vi "Auswertung Registerkarte.vi"(0 "GObject (Eingang)":refnum<vi>, 5 "ClassID":u32, 7 "all rows":string[][](array[string]), 9 "Sprachauswahl":u32, 11 "Fehler (Eingang, kein Fehler)":errorcluster) -> (4 "Clusterelemente":refnum<vi>[](array[refnum]), 15 "error out":errorcluster caption="Fehler (Ausgang)")   [LabVIEW 2015, in "Sprachverwaltung.lvlib"]
uses:
  Sprachverwaltung.lvlib
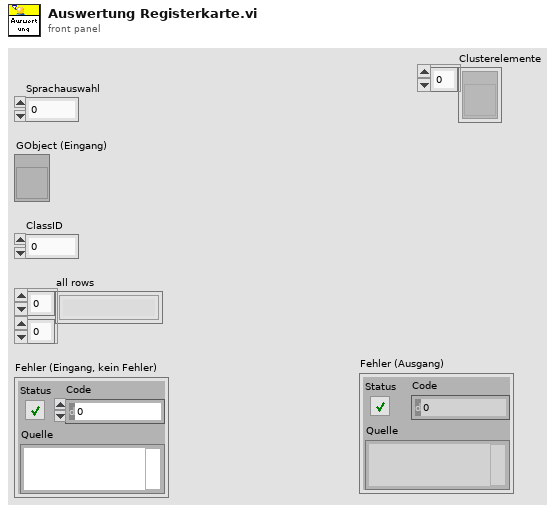
[diagram p1: front panel]
types:
  T1 = typedef "LVStringsAndValuesArrayTypeDef.ctl" = cluster{"String":string, "Value":ext}[]
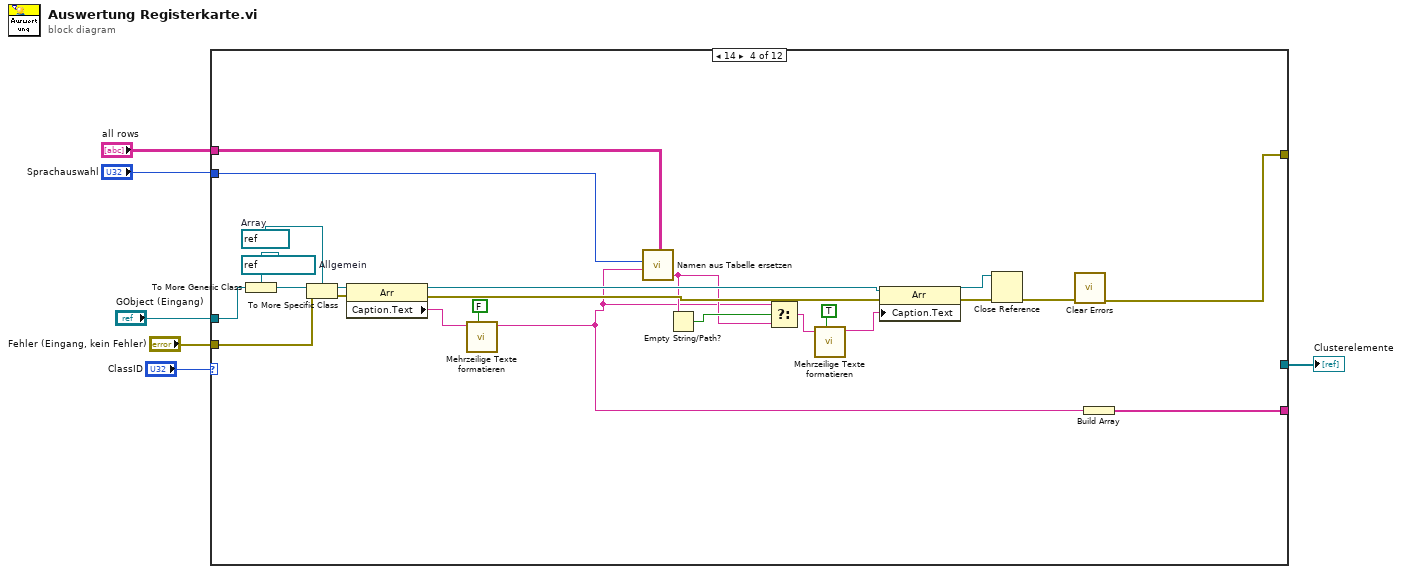
[diagram p0: block diagram]
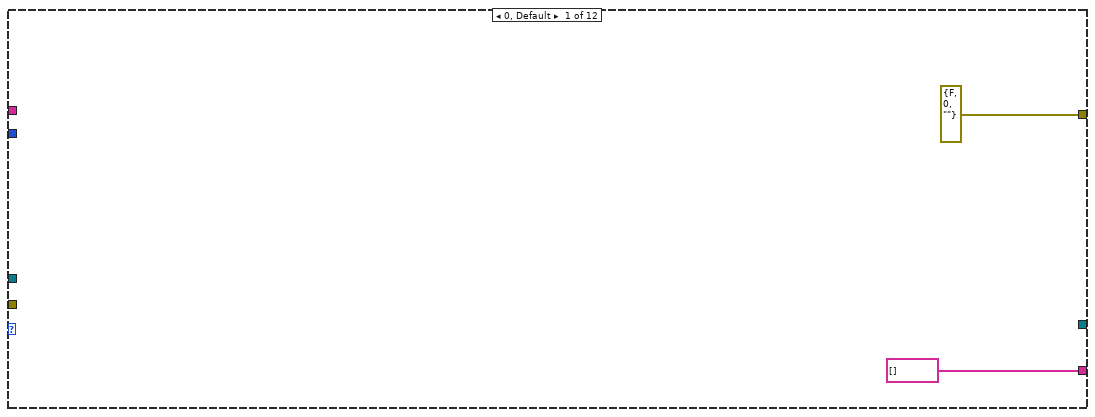
[diagram p2: hidden frame]
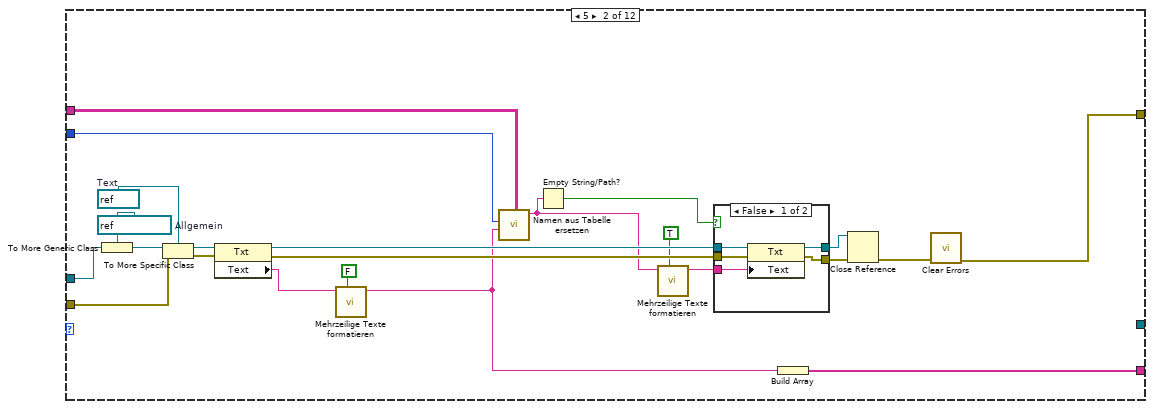
[diagram p3: hidden frame]
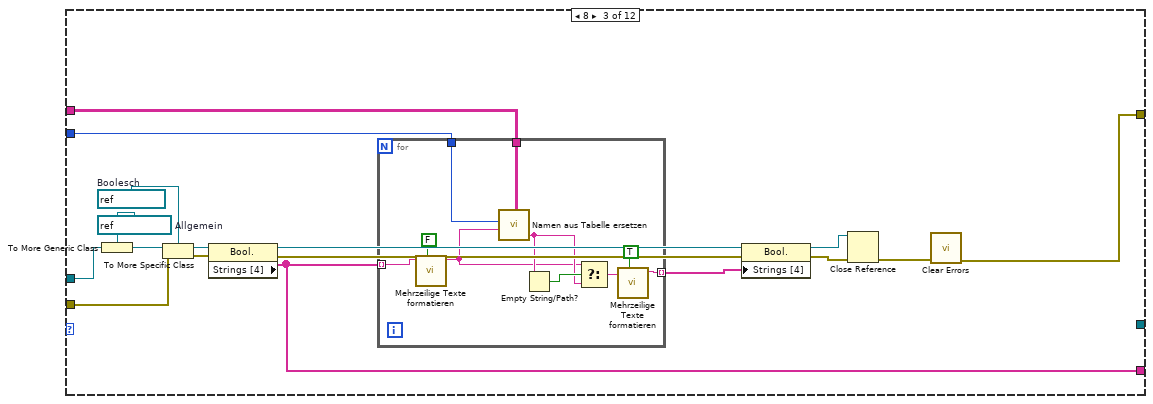
[diagram p5: hidden frame]
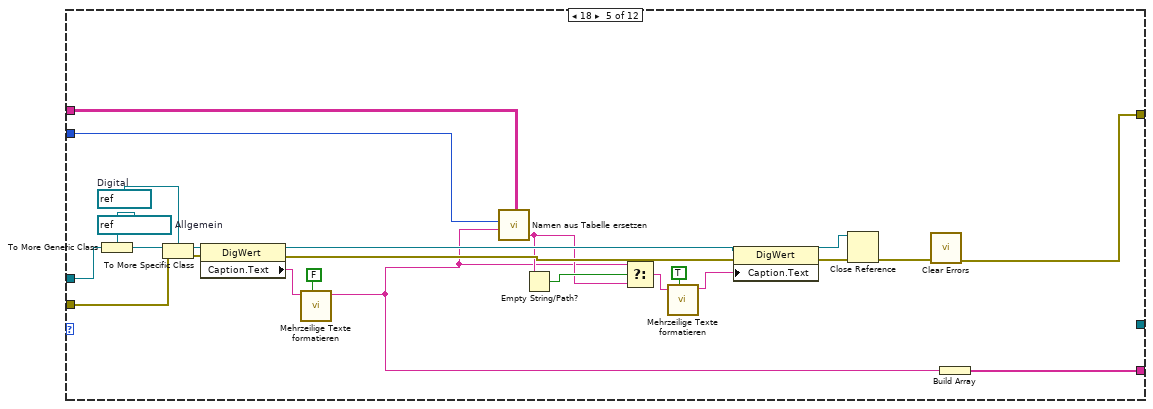
[diagram p6: hidden frame]
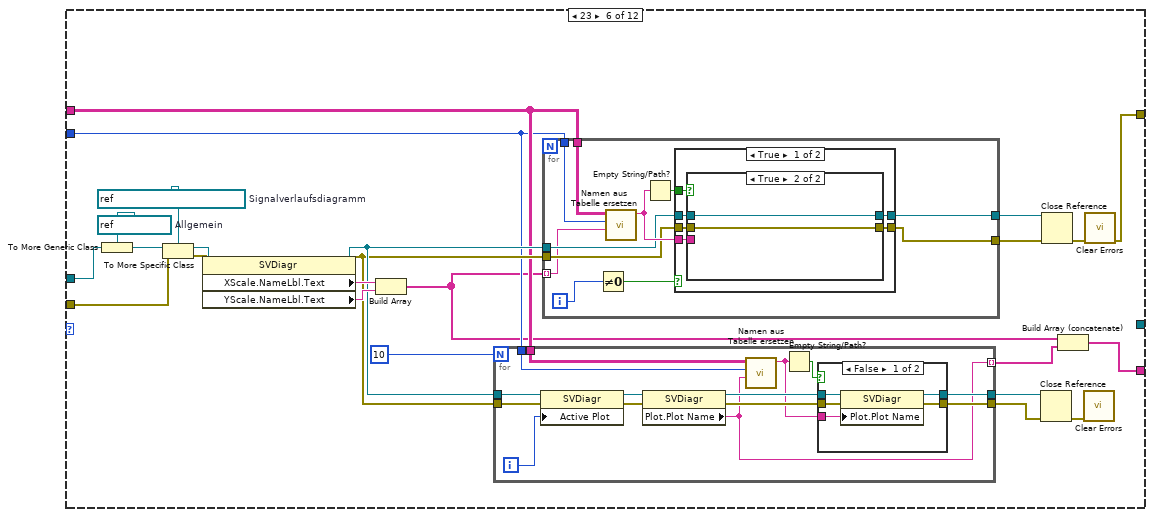
[diagram p7: hidden frame]
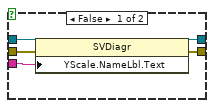
[diagram p9: hidden frame]
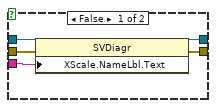
[diagram p11: hidden frame]
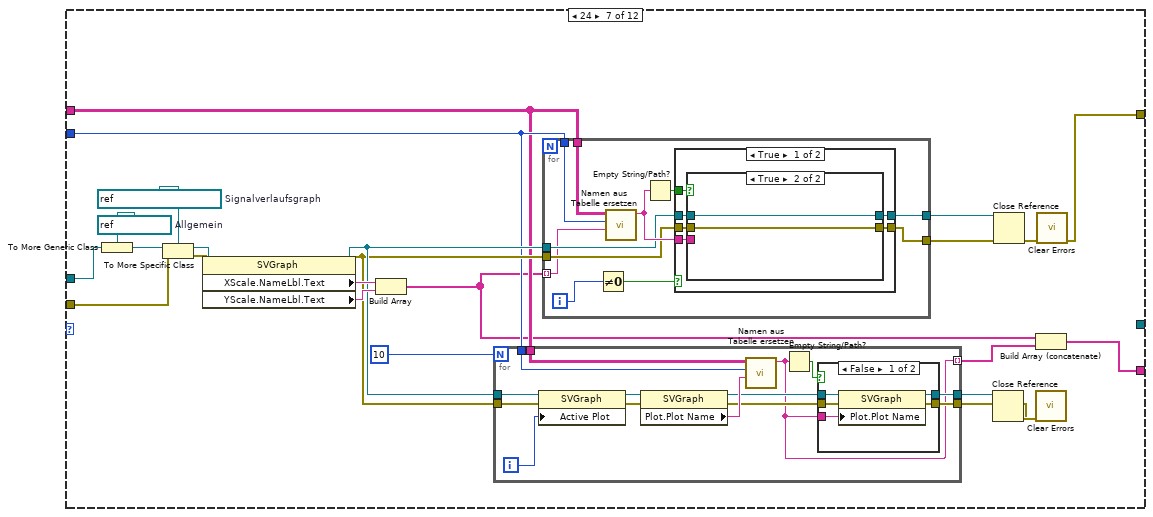
[diagram p12: hidden frame]
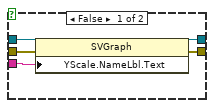
[diagram p14: hidden frame]
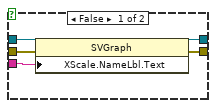
[diagram p16: hidden frame]
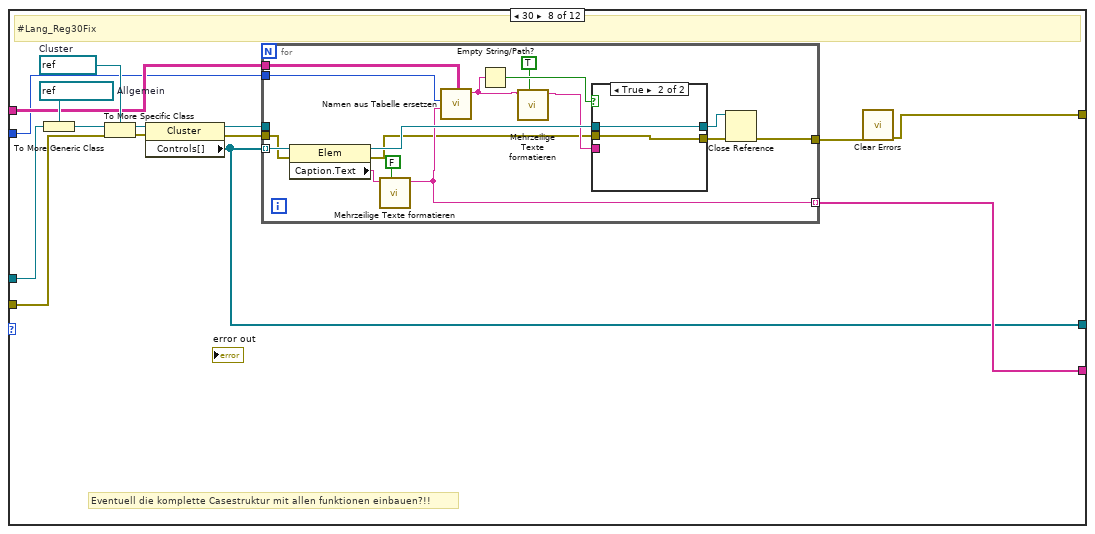
[diagram p17: hidden frame]
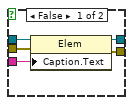
[diagram p18: hidden frame]
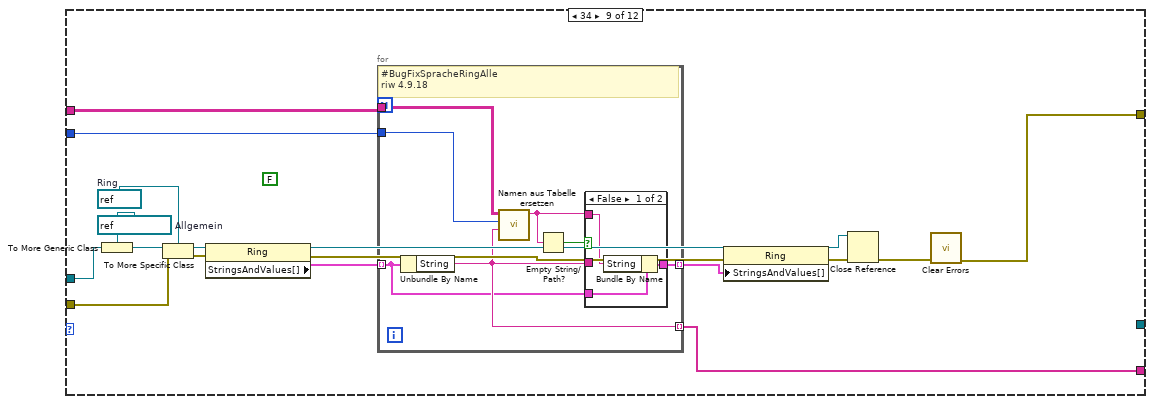
[diagram p19: hidden frame]
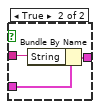
[diagram p20: hidden frame]
diagram:
  n1 = case shown="14" "ClassID" {
    tunnel: "GObject (Eingang)" -> [_ w31 w55 w89 w113 w137 w219 w292 w333 w372 w386 w443]
    tunnel: "Fehler (Eingang, kein Fehler)" -> [_ w28 w52 w86 w110 w134 w216 w289 w330 w369 w387 w440]
    tunnel: "all rows" -> [_ w24 w50 w82 w106 w122 w200 w285 w325 w361 w389 w428]
    tunnel: "Sprachauswahl" -> [_ w17 w49 w81 w105 w121 w204 w284 w324 w360 w388 w420]
    tunnel: [string[] [] ("Strings [4]") w16 w42 w74 w98 w115 w197 w283 w318 w348 w390 w422] -> _
    tunnel: [errorcluster {"status"=FALSE, "code"=0, "source"=""} ("error out") w15 w41 w75 w99 w114 w196 w279 w317 w347 w385 w421] -> _
    tunnel: [_ _ _ _ _ _ _ w278 _ _ _ _] -> w1
    frame 0, Default {
    }
    frame 5 {
      w27 = refnum<vi> refnum  # Text
      w30 = refnum<vi> refnum  # Allgemein
      n2 = To More Generic Class(target class=w30, reference=w31) -> (generic class reference=w29:refnum<vi>)
      n3 = To More Specific Class(target class=w27, reference=w29, error in=w28) -> (specific class reference=w26:refnum<vi>, error out=w25:errorcluster)
      n4 = property class="Txt"(reference=w26, error in=w25) -> (reference out=w22:refnum<vi>, error out=w23:errorcluster, "Text"=w14:string)
      n5 = call "Mehrzeilige Texte formatieren.vi"("Zurück formatieren"=FALSE, "string"=w14) -> ("result string"=w13:string)  [unwired: 9 in]
      n6 = call "Namen aus Tabelle ersetzen.vi"("Regulärer Ausdruck"=w13, "Sprachauswahl"=w17, "Tabelle"=w24) -> ("Übersetzung"=w10:string)  [unwired: 8 in]
      n7 = Empty String/Path?(string/path=w10) -> (empty?=w18:bool)
      n8 = call "Mehrzeilige Texte formatieren.vi"("Zurück formatieren"=TRUE, "string"=w10) -> ("result string"=w9:string)  [unwired: 9 in]
      n9 = case shown="False" w18 {
        tunnel: w23 -> [w36 w37]
        tunnel: w22 -> [w35 w38]
        tunnel: w9 -> [w34 _]
        tunnel: [w33 w37] -> w21
        tunnel: [w32 w38] -> w20
        frame False {
          n10 = property class="Txt"(reference=w35, error in=w36, "Text"=w34) -> (reference out=w32:refnum<vi>, error out=w33:errorcluster)
        }
        frame True {
        }
      }
      n11 = Build Array(w13) -> (w16:string[])
      n12 = Close Reference(reference=w20, error in (no error)=w21) -> (error out=w19:errorcluster)
      n13 = call <vilib>:"Clear Errors.vi"("error in (no error)"=w19) -> ("error out"=w15:errorcluster)  [unwired: 5 in, 1 out]
    }
    frame 8 {
      w51 = refnum<vi> refnum  # Boolesch
      w54 = refnum<vi> refnum  # Allgemein
      n14 = To More Generic Class(target class=w54, reference=w55) -> (generic class reference=w53:refnum<vi>)
      n15 = To More Specific Class(target class=w51, reference=w53, error in=w52) -> (specific class reference=w39:refnum<vi>, error out=w40:errorcluster)
      n16 = property class="Bool."(reference=w39, error in=w40) -> (reference out=w47:refnum<vi>, error out=w48:errorcluster, "Strings [4]"=w42:string[])
      n17 = for {
        tunnel: w42 -> [w60] mode=indexing
        tunnel: w50 -> [w65]
        tunnel: w49 -> [w64]
        tunnel: [w56] -> w43 mode=indexing
        n18 = call "Mehrzeilige Texte formatieren.vi"("Zurück formatieren"=FALSE, "string"=w60) -> ("result string"=w59:string)  [unwired: 9 in]
        n19 = call "Namen aus Tabelle ersetzen.vi"("Regulärer Ausdruck"=w59, "Sprachauswahl"=w64, "Tabelle"=w65) -> ("Übersetzung"=w62:string)  [unwired: 8 in]
        n20 = Empty String/Path?(string/path=w62) -> (empty?=w63:bool)
        n21 = Select(t=w59, s=w63, f=w62) -> (s? t:f=w57:string)
        n22 = call "Mehrzeilige Texte formatieren.vi"("Zurück formatieren"=TRUE, "string"=w57) -> ("result string"=w56:string)  [unwired: 9 in]
      }
      n23 = property class="Bool."(reference=w47, error in=w48, "Strings [4]"=w43) -> (reference out=w45:refnum<vi>, error out=w46:errorcluster)
      n24 = Close Reference(reference=w45, error in (no error)=w46) -> (error out=w44:errorcluster)
      n25 = call <vilib>:"Clear Errors.vi"("error in (no error)"=w44) -> ("error out"=w41:errorcluster)  [unwired: 5 in, 1 out]
    }
    frame 14 {
      w85 = refnum<vi> refnum  # Array
      w88 = refnum<vi> refnum  # Allgemein
      n26 = To More Generic Class(target class=w88, reference=w89) -> (generic class reference=w87:refnum<vi>)
      n27 = To More Specific Class(target class=w85, reference=w87, error in=w86) -> (specific class reference=w84:refnum<vi>, error out=w83:errorcluster)
      n28 = property class="Arr"(reference=w84, error in=w83) -> (reference out=w79:refnum<vi>, error out=w80:errorcluster, "Caption.Text"=w70:string)
      n29 = call "Mehrzeilige Texte formatieren.vi"("Zurück formatieren"=FALSE, "string"=w70) -> ("result string"=w69:string)  [unwired: 9 in]
      n30 = call "Namen aus Tabelle ersetzen.vi"("Regulärer Ausdruck"=w69, "Sprachauswahl"=w81, "Tabelle"=w82) -> ("Übersetzung"=w72:string)  [unwired: 8 in]
      n31 = Empty String/Path?(string/path=w72) -> (empty?=w73:bool)
      n32 = Select(t=w69, s=w73, f=w72) -> (s? t:f=w67:string)
      n33 = call "Mehrzeilige Texte formatieren.vi"("Zurück formatieren"=TRUE, "string"=w67) -> ("result string"=w66:string)  [unwired: 9 in]
      n34 = property class="Arr"(reference=w79, error in=w80, "Caption.Text"=w66) -> (reference out=w77:refnum<vi>, error out=w78:errorcluster)
      n35 = Close Reference(reference=w77, error in (no error)=w78) -> (error out=w76:errorcluster)
      n36 = call <vilib>:"Clear Errors.vi"("error in (no error)"=w76) -> ("error out"=w75:errorcluster)  [unwired: 5 in, 1 out]
      n37 = Build Array(w69) -> (w74:string[])
    }
    frame 18 {
      w109 = refnum<vi> refnum  # Digital
      w112 = refnum<vi> refnum  # Allgemein
      n38 = To More Generic Class(target class=w112, reference=w113) -> (generic class reference=w111:refnum<vi>)
      n39 = To More Specific Class(target class=w109, reference=w111, error in=w110) -> (specific class reference=w108:refnum<vi>, error out=w107:errorcluster)
      n40 = property class="DigWert"(reference=w108, error in=w107) -> (reference out=w103:refnum<vi>, error out=w104:errorcluster, "Caption.Text"=w94:string)
      n41 = call "Mehrzeilige Texte formatieren.vi"("Zurück formatieren"=FALSE, "string"=w94) -> ("result string"=w93:string)  [unwired: 9 in]
      n42 = call "Namen aus Tabelle ersetzen.vi"("Regulärer Ausdruck"=w93, "Sprachauswahl"=w105, "Tabelle"=w106) -> ("Übersetzung"=w96:string)  [unwired: 8 in]
      n43 = Empty String/Path?(string/path=w96) -> (empty?=w97:bool)
      n44 = Select(t=w93, s=w97, f=w96) -> (s? t:f=w91:string)
      n45 = call "Mehrzeilige Texte formatieren.vi"("Zurück formatieren"=TRUE, "string"=w91) -> ("result string"=w90:string)  [unwired: 9 in]
      n46 = property class="DigWert"(reference=w103, error in=w104, "Caption.Text"=w90) -> (reference out=w101:refnum<vi>, error out=w102:errorcluster)
      n47 = Close Reference(reference=w101, error in (no error)=w102) -> (error out=w100:errorcluster)
      n48 = call <vilib>:"Clear Errors.vi"("error in (no error)"=w100) -> ("error out"=w99:errorcluster)  [unwired: 5 in, 1 out]
      n49 = Build Array(w93) -> (w98:string[])
    }
    frame 23 {
      w133 = refnum<vi> refnum  # Signalverlaufsdiagramm
      w136 = refnum<vi> refnum  # Allgemein
      n50 = To More Generic Class(target class=w136, reference=w137) -> (generic class reference=w135:refnum<vi>)
      n51 = To More Specific Class(target class=w133, reference=w135, error in=w134) -> (specific class reference=w132:refnum<vi>, error out=w131:errorcluster)
      n52 = property class="SVDiagr"(reference=w132, error in=w131) -> (reference out=w127:refnum<vi>, error out=w125:errorcluster, "XScale.NameLbl.Text"=w130:string, "YScale.NameLbl.Text"=w129:string)
      n53 = Build Array(w130, w129) -> (w117:string[])
      n54 = for {
        N: 10 -> [_]
        tunnel: w127 -> [w151]
        tunnel: w125 -> [w147]
        tunnel: w122 -> [w146]
        tunnel: w121 -> [w145]
        tunnel: [w141] -> w119
        tunnel: [w140] -> w118
        tunnel: [w138] -> w116 mode=indexing
        i -> [w150]
        n55 = property class="SVDiagr"(reference=w151, error in=w147, "Active Plot"=w150) -> (reference out=w149:refnum<vi>, error out=w148:errorcluster)
        n56 = property class="SVDiagr"(reference=w149, error in=w148) -> (reference out=w144:refnum<vi>, error out=w143:errorcluster, "Plot.Plot Name"=w138:string)
        n57 = call "Namen aus Tabelle ersetzen.vi"("Regulärer Ausdruck"=w138, "Sprachauswahl"=w145, "Tabelle"=w146) -> ("Übersetzung"=w139:string)  [unwired: 8 in]
        n58 = Empty String/Path?(string/path=w139) -> (empty?=w142:bool)
        n59 = case shown="False" w142 {
          tunnel: w144 -> [w156 w158]
          tunnel: w143 -> [w155 w157]
          tunnel: [w154 w158] -> w141
          tunnel: [w153 w157] -> w140
          tunnel: w139 -> [w152 _]
          frame False {
            n60 = property class="SVDiagr"(reference=w156, error in=w155, "Plot.Plot Name"=w152) -> (reference out=w154:refnum<vi>, error out=w153:errorcluster)
          }
          frame True {
          }
        }
      }
      n61 = for {
        tunnel: w122 -> [w169]
        tunnel: w121 -> [w160]
        tunnel: w117 -> [w159] mode=indexing
        tunnel: w127 -> [w164]
        tunnel: w125 -> [w163]
        tunnel: [w162] -> w124
        tunnel: [w161] -> w123
        i -> [w166]
        n62 = Not Equal To 0?(x=w166) -> (x != 0?=w165:bool)
        n63 = call "Namen aus Tabelle ersetzen.vi"("Regulärer Ausdruck"=w159, "Sprachauswahl"=w160, "Tabelle"=w169) -> ("Übersetzung"=w167:string)  [unwired: 8 in]
        n64 = Empty String/Path?(string/path=w167) -> (empty?=w168:bool)
        n65 = case shown="True" w165 {
          tunnel: w168 -> [w175 w188]
          tunnel: w167 -> [w174 w187]
          tunnel: w164 -> [w173 w186]
          tunnel: w163 -> [w172 w185]
          tunnel: [w171 w183] -> w161
          tunnel: [w170 w184] -> w162
          frame True {
            n66 = case shown="True" w175 {
              tunnel: w172 -> [w180 w181]
              tunnel: w173 -> [w179 w182]
              tunnel: [w178 w181] -> w171
              tunnel: [w177 w182] -> w170
              tunnel: w174 -> [w176 _]
              frame False {
                n67 = property class="SVDiagr"(reference=w179, error in=w180, "YScale.NameLbl.Text"=w176) -> (reference out=w177:refnum<vi>, error out=w178:errorcluster)
              }
              frame True {
              }
            }
          }
          frame False {
            n68 = case shown="True" w188 {
              tunnel: w185 -> [w193 w194]
              tunnel: w186 -> [w192 w195]
              tunnel: [w191 w194] -> w183
              tunnel: [w190 w195] -> w184
              tunnel: w187 -> [w189 _]
              frame False {
                n69 = property class="SVDiagr"(reference=w192, error in=w193, "XScale.NameLbl.Text"=w189) -> (reference out=w190:refnum<vi>, error out=w191:errorcluster)
              }
              frame True {
              }
            }
          }
        }
      }
      n70 = Close Reference(reference=w119, error in (no error)=w118) -> (error out=w120:errorcluster)
      n71 = Close Reference(reference=w124, error in (no error)=w123) -> (error out=w128:errorcluster)
      n72 = Build Array (concatenate)(w117, w116) -> (w115:string[])
      n73 = call <vilib>:"Clear Errors.vi"("error in (no error)"=w120) -> ()  [unwired: 5 in, 2 out]
      n74 = call <vilib>:"Clear Errors.vi"("error in (no error)"=w128) -> ("error out"=w114:errorcluster)  [unwired: 5 in, 1 out]
    }
    frame 24 {
      w215 = refnum<vi> refnum  # Signalverlaufsgraph
      w218 = refnum<vi> refnum  # Allgemein
      n75 = To More Generic Class(target class=w218, reference=w219) -> (generic class reference=w217:refnum<vi>)
      n76 = To More Specific Class(target class=w215, reference=w217, error in=w216) -> (specific class reference=w214:refnum<vi>, error out=w213:errorcluster)
      n77 = property class="SVGraph"(reference=w214, error in=w213) -> (reference out=w209:refnum<vi>, error out=w207:errorcluster, "XScale.NameLbl.Text"=w212:string, "YScale.NameLbl.Text"=w211:string)
      n78 = Build Array(w212, w211) -> (w199:string[])
      n79 = for {
        N: 10 -> [_]
        tunnel: w209 -> [w233]
        tunnel: w207 -> [w229]
        tunnel: w200 -> [w228]
        tunnel: w204 -> [w227]
        tunnel: [w222] -> w202
        tunnel: [w221] -> w201
        tunnel: [w220] -> w198 mode=indexing
        i -> [w232]
        n80 = property class="SVGraph"(reference=w233, error in=w229, "Active Plot"=w232) -> (reference out=w231:refnum<vi>, error out=w230:errorcluster)
        n81 = property class="SVGraph"(reference=w231, error in=w230) -> (reference out=w225:refnum<vi>, error out=w224:errorcluster, "Plot.Plot Name"=w226:string)
        n82 = call "Namen aus Tabelle ersetzen.vi"("Regulärer Ausdruck"=w226, "Sprachauswahl"=w227, "Tabelle"=w228) -> ("Übersetzung"=w220:string)  [unwired: 8 in]
        n83 = Empty String/Path?(string/path=w220) -> (empty?=w223:bool)
        n84 = case shown="False" w223 {
          tunnel: w225 -> [w238 w240]
          tunnel: w224 -> [w237 w239]
          tunnel: [w236 w240] -> w222
          tunnel: [w235 w239] -> w221
          tunnel: w220 -> [w234 _]
          frame False {
            n85 = property class="SVGraph"(reference=w238, error in=w237, "Plot.Plot Name"=w234) -> (reference out=w236:refnum<vi>, error out=w235:errorcluster)
          }
          frame True {
          }
        }
      }
      n86 = for {
        tunnel: w200 -> [w251]
        tunnel: w204 -> [w242]
        tunnel: w199 -> [w241] mode=indexing
        tunnel: w209 -> [w246]
        tunnel: w207 -> [w245]
        tunnel: [w244] -> w206
        tunnel: [w243] -> w205
        i -> [w248]
        n87 = Not Equal To 0?(x=w248) -> (x != 0?=w247:bool)
        n88 = call "Namen aus Tabelle ersetzen.vi"("Regulärer Ausdruck"=w241, "Sprachauswahl"=w242, "Tabelle"=w251) -> ("Übersetzung"=w249:string)  [unwired: 8 in]
        n89 = Empty String/Path?(string/path=w249) -> (empty?=w250:bool)
        n90 = case shown="True" w247 {
          tunnel: w250 -> [w257 w270]
          tunnel: w249 -> [w256 w269]
          tunnel: w246 -> [w255 w268]
          tunnel: w245 -> [w254 w267]
          tunnel: [w253 w265] -> w243
          tunnel: [w252 w266] -> w244
          frame True {
            n91 = case shown="True" w257 {
              tunnel: w254 -> [w262 w263]
              tunnel: w255 -> [w261 w264]
              tunnel: [w260 w263] -> w253
              tunnel: [w259 w264] -> w252
              tunnel: w256 -> [w258 _]
              frame False {
                n92 = property class="SVGraph"(reference=w261, error in=w262, "YScale.NameLbl.Text"=w258) -> (reference out=w259:refnum<vi>, error out=w260:errorcluster)
              }
              frame True {
              }
            }
          }
          frame False {
            n93 = case shown="True" w270 {
              tunnel: w267 -> [w275 w276]
              tunnel: w268 -> [w274 w277]
              tunnel: [w273 w276] -> w265
              tunnel: [w272 w277] -> w266
              tunnel: w269 -> [w271 _]
              frame False {
                n94 = property class="SVGraph"(reference=w274, error in=w275, "XScale.NameLbl.Text"=w271) -> (reference out=w272:refnum<vi>, error out=w273:errorcluster)
              }
              frame True {
              }
            }
          }
        }
      }
      n95 = Close Reference(reference=w202, error in (no error)=w201) -> (error out=w203:errorcluster)
      n96 = Close Reference(reference=w206, error in (no error)=w205) -> (error out=w210:errorcluster)
      n97 = Build Array (concatenate)(w199, w198) -> (w197:string[])
      n98 = call <vilib>:"Clear Errors.vi"("error in (no error)"=w203) -> ()  [unwired: 5 in, 2 out]
      n99 = call <vilib>:"Clear Errors.vi"("error in (no error)"=w210) -> ("error out"=w196:errorcluster)  [unwired: 5 in, 1 out]
    }
    frame 30 {
      w288 = refnum<vi> refnum  # Cluster
      w291 = refnum<vi> refnum  # Allgemein
      # "Eventuell die komplette Casestruktur mit allen funktionen einbauen?!!"
      # "#Lang_Reg30Fix"
      n100 = To More Generic Class(target class=w291, reference=w292) -> (generic class reference=w290:refnum<vi>)
      n101 = To More Specific Class(target class=w288, reference=w290, error in=w289) -> (specific class reference=w287:refnum<vi>, error out=w286:errorcluster)
      n102 = property class="Cluster"(reference=w287, error in=w286) -> (reference out=w282:refnum<vi>, error out=w281:errorcluster, "Controls[]"=w278:refnum<vi>[])
      n103 = for {
        tunnel: w285 -> [w308]
        tunnel: w281 -> [w294]
        tunnel: w282 -> [_]
        tunnel: w284 -> [w304]
        tunnel: w278 -> [w303] mode=indexing
        tunnel: [w297] -> w283 mode=indexing
        tunnel: [w301] -> w280
        n104 = property class="Elem"(reference=w303, error in=w294) -> (reference out=w302:refnum<vi>, error out=w293:errorcluster, "Caption.Text"=w298:string)
        n105 = call "Mehrzeilige Texte formatieren.vi"("Zurück formatieren"=FALSE, "string"=w298) -> ("result string"=w297:string)  [unwired: 9 in]
        n106 = call "Namen aus Tabelle ersetzen.vi"("Regulärer Ausdruck"=w297, "Sprachauswahl"=w304, "Tabelle"=w308) -> ("Übersetzung"=w296:string)  [unwired: 8 in]
        n107 = Empty String/Path?(string/path=w296) -> (empty?=w305:bool)
        n108 = call "Mehrzeilige Texte formatieren.vi"("Zurück formatieren"=TRUE, "string"=w296) -> ("result string"=w295:string)  [unwired: 9 in]
        n109 = case shown="True" w305 {
          tunnel: w293 -> [w313 w314]
          tunnel: w302 -> [w312 w315]
          tunnel: w295 -> [w311 _]
          tunnel: [w310 w314] -> w307
          tunnel: [w309 w315] -> w306
          frame False {
            n110 = property class="Elem"(reference=w312, error in=w313, "Caption.Text"=w311) -> (reference out=w309:refnum<vi>, error out=w310:errorcluster)
          }
          frame True {
          }
        }
        n111 = Close Reference(reference=w306, error in (no error)=w307) -> (error out=w301:errorcluster)
      }
      n112 = call <vilib>:"Clear Errors.vi"("error in (no error)"=w280) -> ("error out"=w279:errorcluster)  [unwired: 5 in, 1 out]
    }
    frame 34 {
      (unwired) FALSE
      w329 = refnum<vi> refnum  # Ring
      w332 = refnum<vi> refnum  # Allgemein
      n113 = To More Generic Class(target class=w332, reference=w333) -> (generic class reference=w331:refnum<vi>)
      n114 = To More Specific Class(target class=w329, reference=w331, error in=w330) -> (specific class reference=w328:refnum<vi>, error out=w327:errorcluster)
      n115 = property class="Ring"(reference=w328, error in=w327) -> (reference out=w322:refnum<vi>, error out=w323:errorcluster, "StringsAndValues[]"=w326:T1)
      n116 = for {
        tunnel: w326 -> [w335] mode=indexing
        tunnel: w325 -> [w340]
        tunnel: w324 -> [w339]
        tunnel: [w336] -> w318 mode=indexing
        tunnel: [w334] -> w316 mode=indexing
        # "#BugFixSpracheRingAlle\nriw 4.9.18"
        n117 = Unbundle By Name(w335) -> ("String"=w336:string)
        n118 = call "Namen aus Tabelle ersetzen.vi"("Regulärer Ausdruck"=w336, "Sprachauswahl"=w339, "Tabelle"=w340) -> ("Übersetzung"=w337:string)  [unwired: 8 in]
        n119 = Empty String/Path?(string/path=w337) -> (empty?=w338:bool)
        n120 = case shown="False" w338 {
          tunnel: w335 -> [w343 w346]
          tunnel: w337 -> [w342 _]
          tunnel: [w341 w345] -> w334
          tunnel: w336 -> [_ w344]
          frame False {
            n121 = Bundle By Name(cluster=w343, "String"=w342) -> (w341:cluster{"String":string, "Value":ext})
          }
          frame True {
            n122 = Bundle By Name(cluster=w346, "String"=w344) -> (w345:cluster{"String":string, "Value":ext})
          }
        }
      }
      n123 = property class="Ring"(reference=w322, error in=w323, "StringsAndValues[]"=w316) -> (reference out=w320:refnum<vi>, error out=w321:errorcluster)
      n124 = Close Reference(reference=w320, error in (no error)=w321) -> (error out=w319:errorcluster)
      n125 = call <vilib>:"Clear Errors.vi"("error in (no error)"=w319) -> ("error out"=w317:errorcluster)  [unwired: 5 in, 1 out]
    }
    frame 46 {
      w368 = refnum<vi> refnum  # MehrspaltigesListenfeld
      w371 = refnum<vi> refnum  # Allgemein
      # "Eventuell die komplette Casestruktur mit allen funktionen einbauen?!!"
      n126 = To More Generic Class(target class=w371, reference=w372) -> (generic class reference=w370:refnum<vi>)
      n127 = To More Specific Class(target class=w368, reference=w370, error in=w369) -> (specific class reference=w362:refnum<vi>, error out=w367:errorcluster)
      n128 = property class="MehrSpaltFeld"(reference=w362, error in=w367) -> (reference out=w364:refnum<vi>, error out=w363:errorcluster, "RowHdrs[]"=w350:string[])
      n129 = property class="MehrSpaltFeld"(reference=w362) -> (reference out=w359:refnum<vi>, error out=w358:errorcluster, "ColHdrString"=w349:string[])  [unwired: 1 in]
      n130 = Build Array (concatenate)(w350, w349) -> (w348:string[])
      n131 = for {
        tunnel: w361 -> [w384]
        tunnel: w360 -> [w383]
        tunnel: w350 -> [w381] mode=indexing
        tunnel: [w379] -> w365 mode=indexing
        n132 = call "Namen aus Tabelle ersetzen.vi"("Regulärer Ausdruck"=w381, "Sprachauswahl"=w383, "Tabelle"=w384) -> ("Übersetzung"=w380:string)  [unwired: 8 in]
        n133 = Empty String/Path?(string/path=w380) -> (empty?=w382:bool)
        n134 = Select(t=w381, s=w382, f=w380) -> (s? t:f=w379:string)
      }
      n135 = for {
        tunnel: w361 -> [w378]
        tunnel: w360 -> [w377]
        tunnel: w349 -> [w373] mode=indexing
        tunnel: [w374] -> w357 mode=indexing
        n136 = call "Namen aus Tabelle ersetzen.vi"("Regulärer Ausdruck"=w373, "Sprachauswahl"=w377, "Tabelle"=w378) -> ("Übersetzung"=w375:string)  [unwired: 8 in]
        n137 = Empty String/Path?(string/path=w375) -> (empty?=w376:bool)
        n138 = Select(t=w373, s=w376, f=w375) -> (s? t:f=w374:string)
      }
      n139 = property class="MehrSpaltFeld"(reference=w359, error in=w358, "ColHdrString"=w357) -> (reference out=w352:refnum<vi>, error out=w354:errorcluster)
      n140 = property class="MehrSpaltFeld"(reference=w364, error in=w363, "RowHdrs[]"=w365) -> (reference out=w351:refnum<vi>, error out=w355:errorcluster)
      n141 = Merge Errors(w355, w354) -> (w353:errorcluster)
      n142 = Close Reference(reference=w351, error in (no error)=w353) -> (error out=w356:errorcluster)
      n143 = Close Reference(reference=w352, error in (no error)=w353) -> (error out=w366:errorcluster)
      n144 = call <vilib>:"Clear Errors.vi"("error in (no error)"=w356) -> ("error out"=w347:errorcluster)  [unwired: 5 in, 1 out]
      n145 = call <vilib>:"Clear Errors.vi"("error in (no error)"=w366) -> ()  [unwired: 5 in, 2 out]
    }
    frame 55 {
      w398 = refnum<vi> refnum  # Registerkartenelement
      w400 = refnum<vi> refnum  # Allgemein
      # "mit RKUntertitel schon - riw 11.07.2018 #BugFixSpracheRegisterkarten"
      # "Funktioniert nicht!!"
      # "rekursiv - daher ablaufinvariant - aber gemeinsam genutzt ! riw"
      n146 = To More Generic Class(target class=w400, reference=w386) -> (generic class reference=w399:refnum<vi>)
      n147 = To More Specific Class(target class=w398, reference=w399, error in=w387) -> (specific class reference=w397:refnum<vi>, error out=w396:errorcluster)
      n148 = property class="RKElem"(reference=w397, error in=w396) -> (error out=w395:errorcluster, "Pages"=w391:refnum<vi>[])  [unwired: 1 out]
      n149 = call "Registerkartenverwaltung.vi"("Sprachauswahl"=w388, "all rows"=w389, "Seiten"=w391) -> ()  [unwired: 9 in]
      n150 = for {
        tunnel: w395 -> [w411]
        tunnel: w391 -> [w410] mode=indexing
        tunnel: w388 -> [w404]
        tunnel: w389 -> [w409]
        tunnel: [w406] -> w394
        tunnel: [w405] -> w393
        tunnel: [w403] -> w390 mode=indexing
        n151 = property class="Seite"(reference=w410, error in=w411) -> (reference out=w402:refnum<vi>, error out=w408:errorcluster, "TabCaption"=w403:string)
        n152 = call "Namen aus Tabelle ersetzen.vi"("Regulärer Ausdruck"=w403, "Sprachauswahl"=w404, "Tabelle"=w409) -> ("Übersetzung"=w407:string)  [unwired: 8 in]
        n153 = Empty String/Path?(string/path=w407) -> (empty?=w401:bool)
        n154 = case shown="False" w401 {
          tunnel: w408 -> [w414 w418]
          tunnel: w402 -> [w417 w419]
          tunnel: [w415 w418] -> w405
          tunnel: [w416 w419] -> w406
          tunnel: w407 -> [w413 _]
          frame False {
            # "#BugFixSpracheRegisterkarten"
            n155 = property class="Seite"(reference=w417, error in=w414, "IndependentLabel"=TRUE ("Unabhängige Beschriftung"), "TabCaption"=w413) -> (reference out=w416:refnum<vi>, error out=w415:errorcluster)
          }
          frame True {
          }
        }
      }
      n156 = Close Reference(reference=w394, error in (no error)=w393) -> (error out=w392:errorcluster)
      n157 = call <vilib>:"Clear Errors.vi"("error in (no error)"=w392) -> ("error out"=w385:errorcluster)  [unwired: 5 in, 1 out]
    }
    frame 83 {
      w439 = refnum<vi> refnum  # XYGraph
      w442 = refnum<vi> refnum  # Allgemein
      n158 = To More Generic Class(target class=w442, reference=w443) -> (generic class reference=w441:refnum<vi>)
      n159 = To More Specific Class(target class=w439, reference=w441, error in=w440) -> (specific class reference=w438:refnum<vi>, error out=w437:errorcluster)
      n160 = property class="XYGraph"(reference=w438, error in=w437) -> (reference out=w433:refnum<vi>, error out=w431:errorcluster, "XScale.NameLbl.Text"=w436:string, "YScale.NameLbl.Text"=w435:string)
      n161 = Build Array(w436, w435) -> (w424:string[])
      n162 = for {
        N: 10 -> [_]
        tunnel: w433 -> [w457]
        tunnel: w431 -> [w453]
        tunnel: w428 -> [w452]
        tunnel: w420 -> [w451]
        tunnel: [w446] -> w426
        tunnel: [w445] -> w425
        tunnel: [w444] -> w423 mode=indexing
        i -> [w456]
        n163 = property class="XYGraph"(reference=w457, error in=w453, "Active Plot"=w456) -> (reference out=w455:refnum<vi>, error out=w454:errorcluster)
        n164 = property class="XYGraph"(reference=w455, error in=w454) -> (reference out=w449:refnum<vi>, error out=w448:errorcluster, "Plot.Plot Name"=w450:string)
        n165 = call "Namen aus Tabelle ersetzen.vi"("Regulärer Ausdruck"=w450, "Sprachauswahl"=w451, "Tabelle"=w452) -> ("Übersetzung"=w444:string)  [unwired: 8 in]
        n166 = Empty String/Path?(string/path=w444) -> (empty?=w447:bool)
        n167 = case shown="True" w447 {
          tunnel: w449 -> [w462 w464]
          tunnel: w448 -> [w461 w463]
          tunnel: [w460 w464] -> w446
          tunnel: [w459 w463] -> w445
          tunnel: w444 -> [w458 _]
          frame False {
            n168 = property class="XYGraph"(reference=w462, error in=w461, "Plot.Plot Name"=w458) -> (reference out=w460:refnum<vi>, error out=w459:errorcluster)
          }
          frame True {
          }
        }
      }
      n169 = for {
        tunnel: w428 -> [w475]
        tunnel: w420 -> [w466]
        tunnel: w424 -> [w465] mode=indexing
        tunnel: w433 -> [w470]
        tunnel: w431 -> [w469]
        tunnel: [w468] -> w430
        tunnel: [w467] -> w429
        i -> [w472]
        n170 = Not Equal To 0?(x=w472) -> (x != 0?=w471:bool)
        n171 = call "Namen aus Tabelle ersetzen.vi"("Regulärer Ausdruck"=w465, "Sprachauswahl"=w466, "Tabelle"=w475) -> ("Übersetzung"=w473:string)  [unwired: 8 in]
        n172 = Empty String/Path?(string/path=w473) -> (empty?=w474:bool)
        n173 = case shown="True" w471 {
          tunnel: w474 -> [w481 w494]
          tunnel: w473 -> [w480 w493]
          tunnel: w470 -> [w479 w492]
          tunnel: w469 -> [w478 w491]
          tunnel: [w477 w489] -> w467
          tunnel: [w476 w490] -> w468
          frame True {
            n174 = case shown="True" w481 {
              tunnel: w478 -> [w486 w487]
              tunnel: w479 -> [w485 w488]
              tunnel: [w484 w487] -> w477
              tunnel: [w483 w488] -> w476
              tunnel: w480 -> [w482 _]
              frame False {
                n175 = property class="XYGraph"(reference=w485, error in=w486, "YScale.NameLbl.Text"=w482) -> (reference out=w483:refnum<vi>, error out=w484:errorcluster)
              }
              frame True {
              }
            }
          }
          frame False {
            n176 = case shown="True" w494 {
              tunnel: w491 -> [w499 w500]
              tunnel: w492 -> [w498 w501]
              tunnel: [w497 w500] -> w489
              tunnel: [w496 w501] -> w490
              tunnel: w493 -> [w495 _]
              frame False {
                n177 = property class="XYGraph"(reference=w498, error in=w499, "XScale.NameLbl.Text"=w495) -> (reference out=w496:refnum<vi>, error out=w497:errorcluster)
              }
              frame True {
              }
            }
          }
        }
      }
      n178 = Close Reference(reference=w426, error in (no error)=w425) -> (error out=w427:errorcluster)
      n179 = Close Reference(reference=w430, error in (no error)=w429) -> (error out=w434:errorcluster)
      n180 = Build Array (concatenate)(w424, w423) -> (w422:string[])
      n181 = call <vilib>:"Clear Errors.vi"("error in (no error)"=w427) -> ()  [unwired: 5 in, 2 out]
      n182 = call <vilib>:"Clear Errors.vi"("error in (no error)"=w434) -> ("error out"=w421:errorcluster)  [unwired: 5 in, 1 out]
    }
  }
  "Clusterelemente" <- w1
